vi "AlliGator Phasor Plot Image ROI Storage [SGL] v3.vi"(7 "Current Phasor Plot ROI Color":u32(colorbox), 8 "Error In":errorcluster, 9 "Current ROI Descriptor":T2 {"Contours"."Type" items=["No Selection", "Point", "Line", "Rectangle", "Oval", "Polygon", "Freehand Region", "Annulus", "Unused2", "Unused3", "Broken Line", "Freehand Line", "Rotated Rectangle"]}, 10 "Default Name (\"ROI\")":string="ROI", 11 "Action":T1=enum."Update Current ROI Descriptor") -> (0 "Error Out":errorcluster, 1 "Current ROI Descriptor":T2 {"Contours"."Type" items=["No Selection", "Point", "Line", "Rectangle", "Oval", "Polygon", "Freehand Region", "Annulus", "Unused2", "Unused3", "Broken Line", "Freehand Line", "Rotated Rectangle"]}, 2 "Current ROI Name":string, 3 "Current Phasor Plot Image ROI Index":i32, 4 "Old ROI Name":string, 5 "Current Phasor Plot ROI Color":u32(colorbox))   [LabVIEW 2021, in "AlliGator ROIs.lvlib"]
doc: "Handles single Phasor Plot image ROI storage."
uses:
  AlliGator ROIs.lvlib
  AlliGator ROI Manager Actions.ctl
  Image/Named ROI Description.ctl
  AlliGator Variables List.ctl
  Variant/Variant to Data/Variant to I32.vi
  GUI/GUI.lvlib
  Image/Image.lvlib
  AlliGator Globals, Variables & Constants.lvlib
  Variant/Variant to Data/Variant to Data.lvlib
  Strings/Strings.lvlib
panel:
  # "see the AlliGator License on the block diagram (Ctrl+E or Window:Show Block Diagram)"
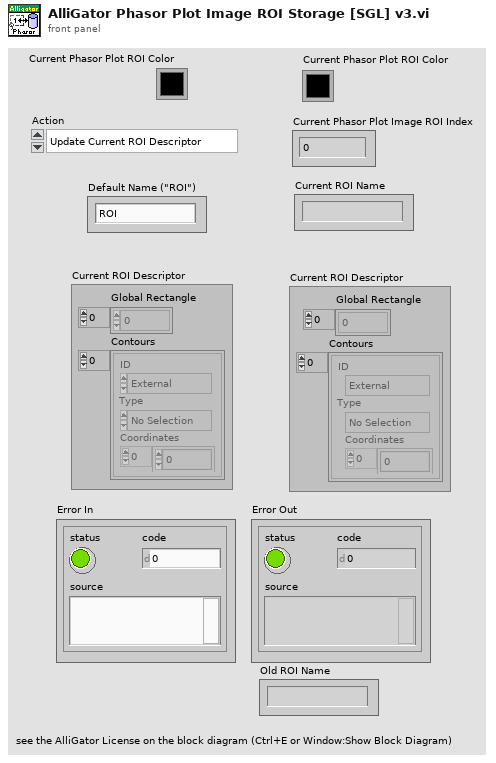
[diagram p1: front panel]
types:
  T1 = typedef "AlliGator ROIs.lvlib/AlliGator ROI Manager Actions.ctl" = enum16{"Undefined", "Delete Current ROI", "Delete All Unselected ROIs", "Delete Multiple ROIs", "Delete All ROIs", "Swap ROIs", "Insert ROI", "Update Current ROI Descriptor", "Rename Current ROI", "Store New ROI", "Store Multiple ROIs", "Select Next ROI", "Select Previous ROI", "Find Selected ROI", "Show All ROIs", "Update ROI Manager Window", "Merge All ROIs", "Unmerge ROI", "Set Selected ROI by ID"}
  T2 = typedef "ROI Descriptor" = cluster{"Global Rectangle":i32[], "Contours":cluster{"ID":enum32{"External", "Internal"}, "Type":u32, "Coordinates":i32[]}[]}
  T3 = typedef "AlliGator Globals, Variables & Constants.lvlib/AlliGator Variables List.ctl" = enum16{"---- GUI ----", "Initialization Status", "State Indicators Refnum", "Original AlliGator Menu Items", "Current Action Loop State", "Script in progress", "Playback", "Loop Playback", "Search ROI Used", "Search ROI", "Decay Graph Max Legend Size", "Intensity Graph Max Legend Size", "Decay Statistics Graph Max Legend Size", "Phasor Graph Max Legend Size", "Phasor Ratio Graph Max Legend Size", "Lifetime Graph Max Legend Size", "---- Files ----", "Export Dataset Frames as Individual Files", "Show Batch Export Help Balloons", "Frames in Dataset", "ptu File Frame Start Indices", "Current Frame in Dataset", "Current Frame Timestamp", "------ Python Plugins ------", "Python Plugins Information", "Python Session", "Valid Python Session?", "---- Source Image ----", "Dataset Loaded", "Dataset Metadata", "Dataset Channel", "Dataset Data Description", "Background Dataset Metadata", "Background Dataset Channel", "Background Dataset Data Description", "Background File Subtraction", "Background File Path", "Background File Pile-up Correction", "Background File Pixel Well Capacity", "Background File Scaling Factor", "Source Image ROIs", "Current Source Image ROI", "Source Image ROI Event Refnum", "X_Source Image Display Range", "X_Source Image Palette Information", "Source Image Palette List", "Source Image Scale", "Current Dataset Load Settings", "Source Image:ROI Overlay Color", "---- Image Profile Window ----", "Image Profile:Overlay ROI in Source Image", "Image Profile Window Event Refnum", "Image Profile:IntensityType", "Image Profile:Intensity Average Type", "Image Profile:Intensity-weighted SDV", "Image Profile:Box Profile Type", "Image Profile Window Open", "Image Profile:Plotted Fit Parameter", "X_Type of Displayed Image", "X_Time Gate Slider", "Dataset Path", "Source Image Overlay to Erase", "Is Displayed Image Accumulated", "White Light Image Modified", "Mask Image Modified", "Macrotime Gate Separation", "------ Phasor Graph -------", "Phasor Graph:Show Line", "---- Phasor Plot ---", "Phasor Plot Parameters Changed", "FLI Dataset Modified since last Phasor Plot Calculation", "Phasor Harmonics Data", "Selected Phasor Harmonics", "Phasor Harmonic Manager Event Refnum", "Phasor Plot ROIs", "Current Phasor Plot ROI", "Phasor Plot ROI Event Refnum", "Phasor Plot Image Reference Points", "Phasor Plot Computed", "Phasor Plot Palette Information", "Phasor Plot Palette List", "Phasor Ratio Palette Information", "Phasor Ratio Palette List", "Phasor Image Scale", "Phasor Plot Image Overlay to Erase", "Phasor Plot Image Elements to Update", "Current Phasor Plot Calculation Parameters", "Current Phasor Calibration Options", "Reset Cumulated Phasor Plot", "Phasor Ratio Reference 1", "Phasor Ratio Lifetime Reference 1", "Phasor Ratio Reference 1 Frequency", "Phasor Ratio Reference 2", "Phasor Ratio Lifetime Reference 2", "Phasor Ratio Reference 2 Frequency", "---- Decay Analysis ----", "Number of Selected Decays to Fit", "LS Fit Results", "LAR Fit Results", "BS Fit Results", "Last Decay Max - Min", "Best Fit Parameters", "Best Fit Parameter Names", "Actual Size X", "Actual Size Y", "Binning X", "Binning Y", "Actual # Gates", "Dataset Number", "Gates to...", "Gates Skipped", "Gates to keep", "Gate Step", "Gate Separation", "Reversed Gates", "Pile-up Correction", "Pixel Well Capacity", "Background Subtracted", "Background Subtraction Method", "Background Definition Range", "Background File (deprecated)", "Number of Dataset Accumulated", "Array of Accumulated Dataset Paths", "Do Averaged Datasets", "Destination File Path", "Process Plot Target", "Use 1/D as Phasor Frequency", "---- Decay Fit Parameter Map -----", "Decay Fit Parameter Map Palette Information", "Decay Fit Parameter Map Palette List", "Local Decay Graph Window Event Refnum", "------- Local Decay Window ---------", "Use normalized IRF for convolution", "----- Miscellaneous ----", "Skippable Dialog Windows Status"}
  T4 = typedef "Image.lvlib/Named ROI Description.ctl" = cluster{"ROI Descriptor":T2, "ROI Name":string, "Overlay Color":u32}
  T5 = typedef "AlliGator ROIs.lvlib/AlliGator Image ROI Event refnum.ctl" = refnum<user-event>
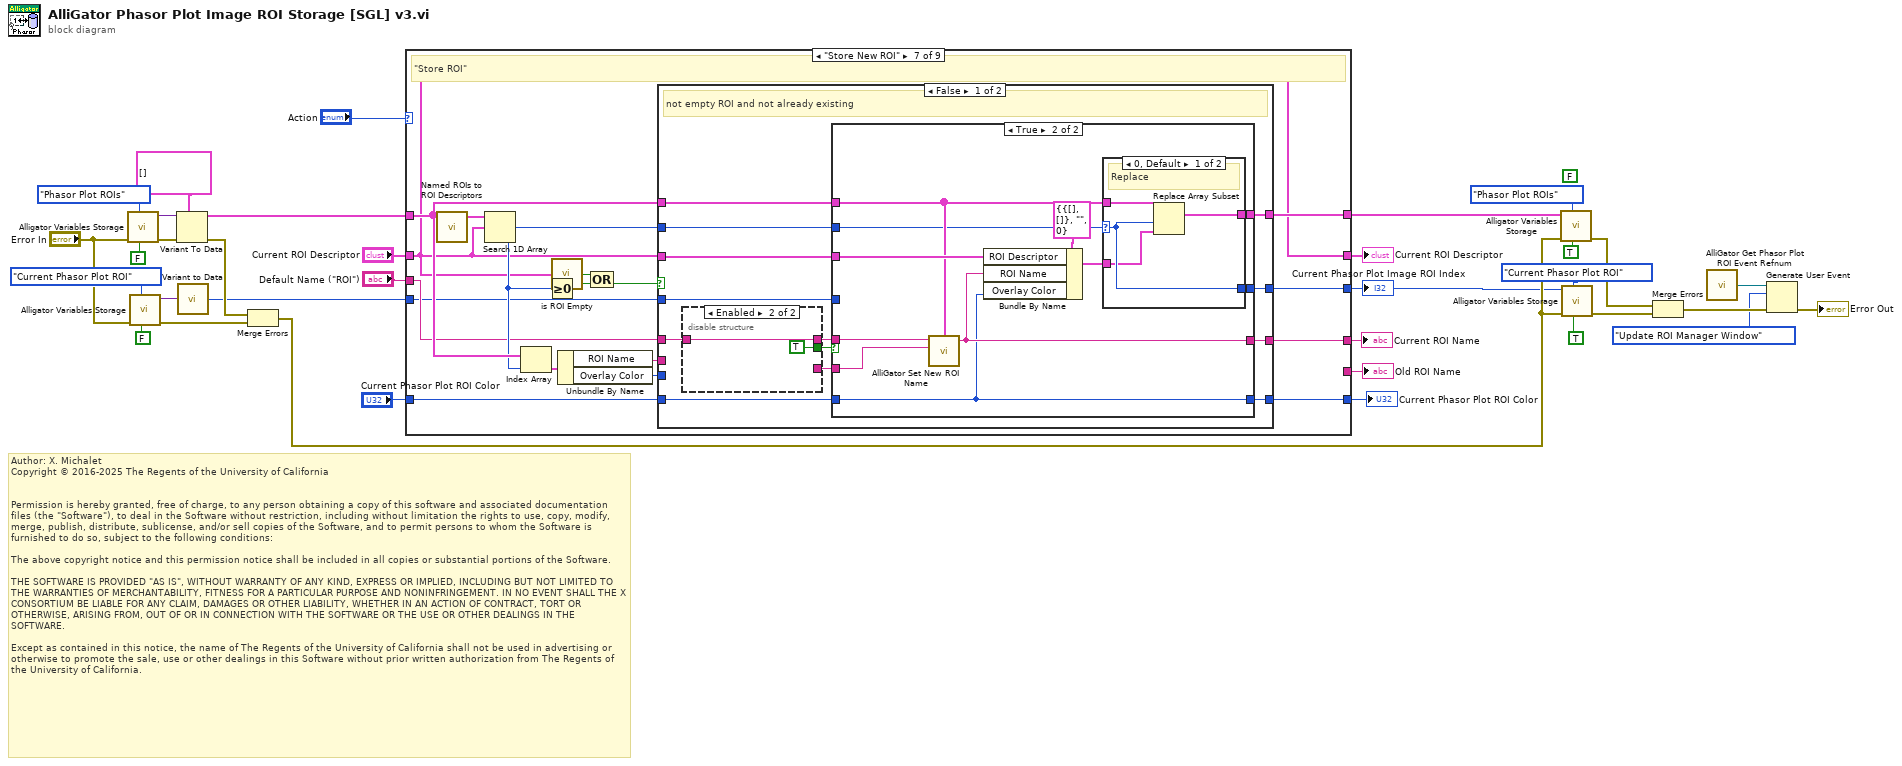
[diagram p0: block diagram]
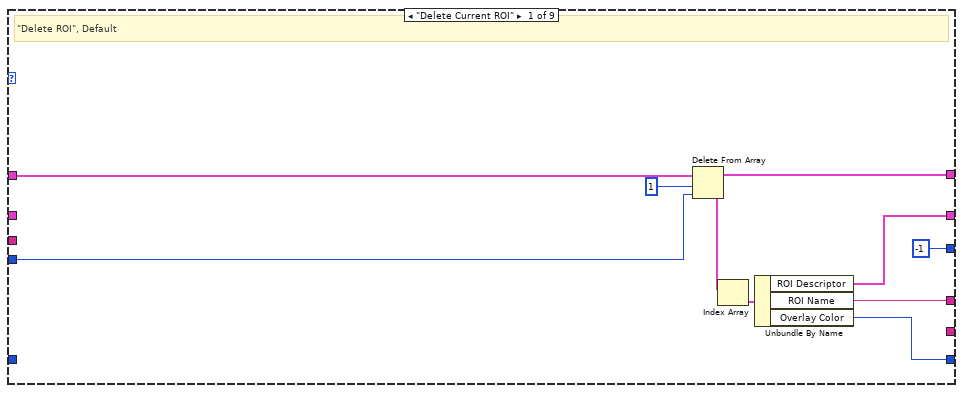
[diagram p2: hidden frame]
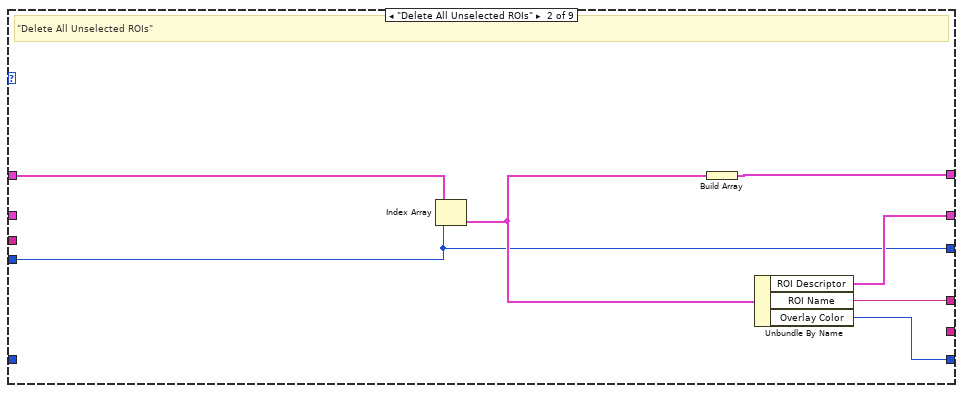
[diagram p3: hidden frame]
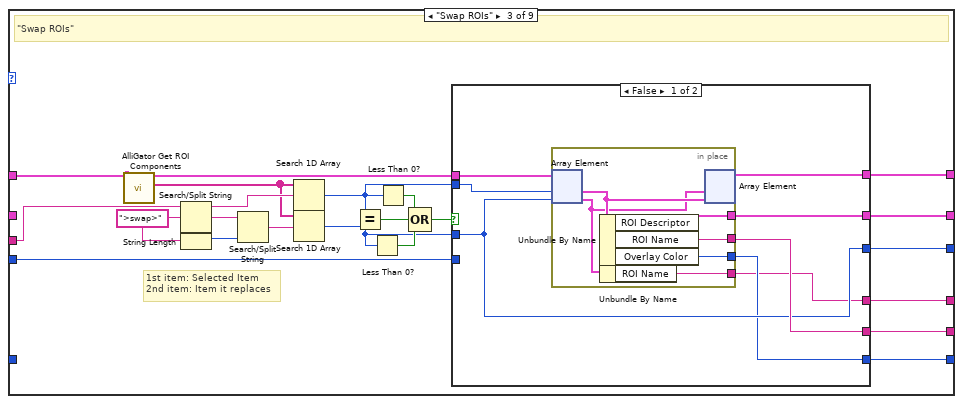
[diagram p4: hidden frame]
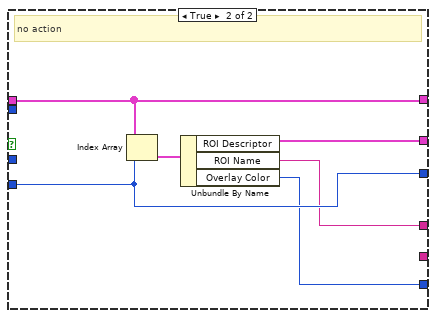
[diagram p5: hidden frame]
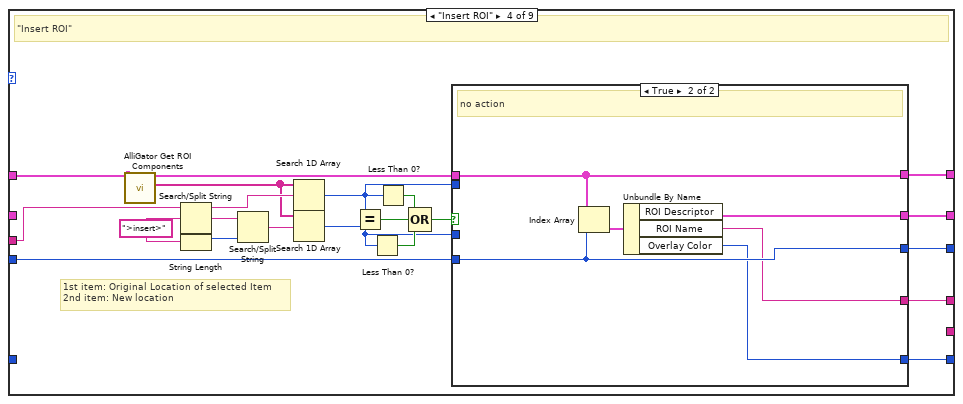
[diagram p6: hidden frame]
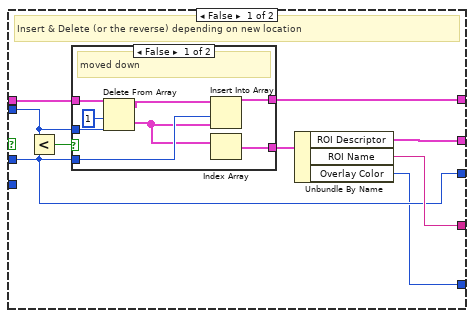
[diagram p7: hidden frame]
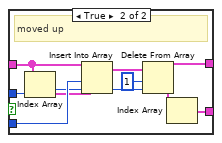
[diagram p8: hidden frame]
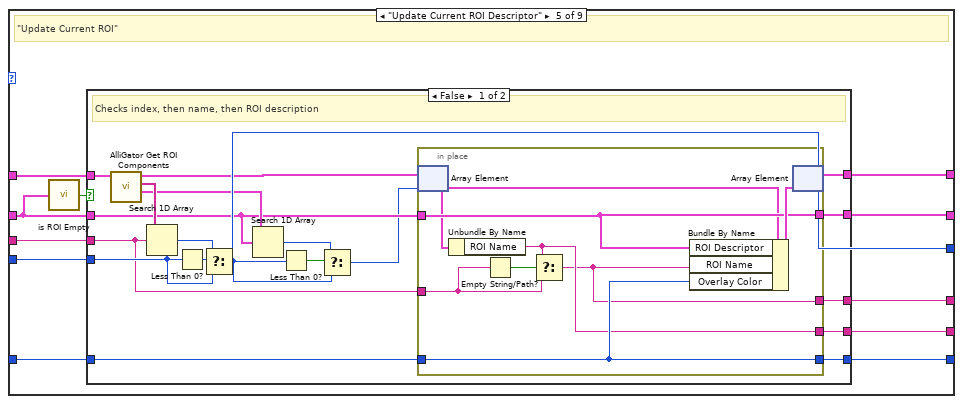
[diagram p9: hidden frame]
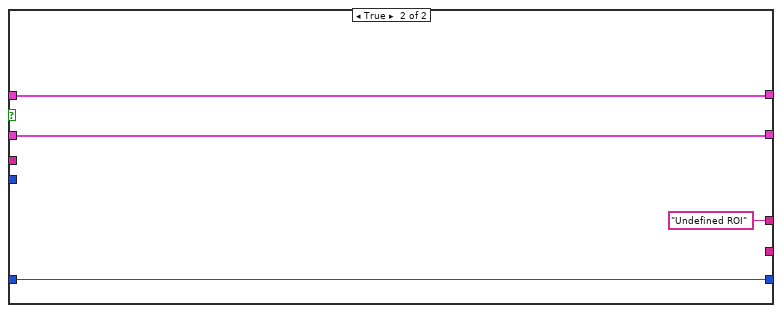
[diagram p10: hidden frame]
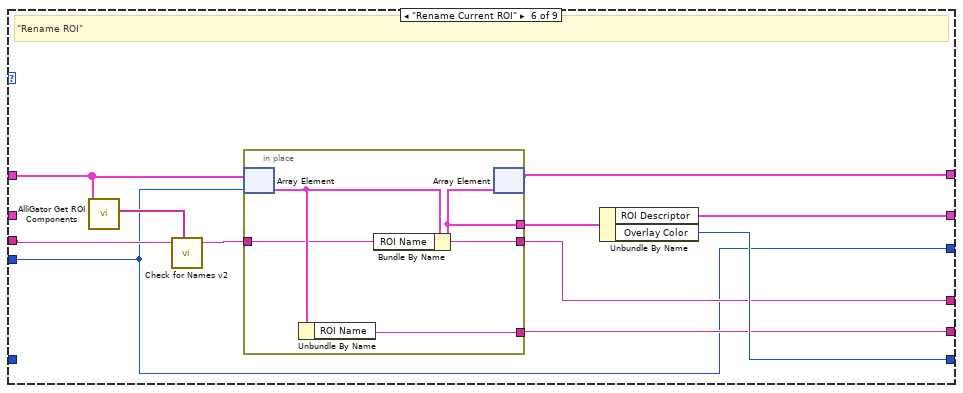
[diagram p11: hidden frame]
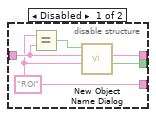
[diagram p12: hidden frame]
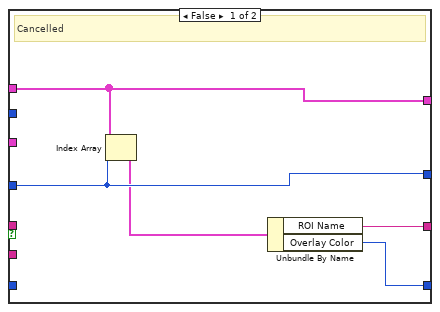
[diagram p13: hidden frame]
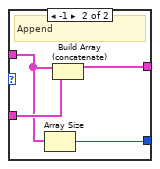
[diagram p14: hidden frame]
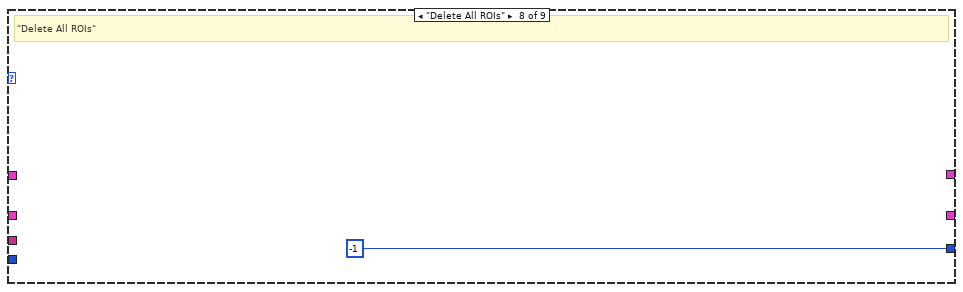
[diagram p16: hidden frame]
diagram:
  (unwired) FALSE ("Get(F)/Set")
  # "Author: X. Michalet\nCopyright © 2016-2025 The Regents of the University of California\n \n\nPermission is hereby granted, free of charge, to any person obtaining a copy of this software and associated documentation files (the \"Software\"), to deal in the Software without restriction, including without limitation the rights to use, copy, modify, merge, publish, distribute, sublicense, and/or sell copies of the Software, and to permit persons to whom the Software is furnished to do so, subject to the following conditions:\n\nThe above copyright notice and this permission notice shall be included in all copies or substantial portions of the Software.\n\nTHE SOFTWARE IS PROVIDED \"AS IS\", WITHOUT WARRANTY OF ANY KIND, EXPRESS OR IMPLIED, INCLUDING BUT NOT LIMITED TO THE WARRANTIES OF MERCHANTABILITY, FITNESS FOR A PARTICULAR PURPOSE AND NONINFRINGEMENT. IN NO EVENT SHALL THE X CONSORTIUM BE LIABLE FOR ANY CLAIM, DAMAGES OR OTHER LIABILITY, WHETHER IN AN ACTION OF CONTRACT, TORT OR OTHERWISE, ARISING FROM, OUT OF OR IN CONNECTION WITH THE SOFTWARE OR THE USE OR OTHER DEALINGS IN THE SOFTWARE.\n\nExcept as contained in this notice, the name of The Regents of the University of California shall not be used in advertising or otherwise to promote the sale, use or other dealings in this Software without prior written authorization from The Regents of the University of California."
  n1 = call "Alligator Variables Storage.vi"("Get(F)/Set"=FALSE, "AlliGator Variable"=AlliGator_Variables_List."Phasor Plot ROIs" ("Alligator Variable"), "Error In"="Error In") -> ("Error Out"=w32:errorcluster, "Data out"=w33:variant)  [unwired: 6 in, 1 out]
  n2 = call "Alligator Variables Storage.vi"("Get(F)/Set"=FALSE, "AlliGator Variable"=AlliGator_Variables_List."Current Phasor Plot ROI" ("Alligator Variable"), "Error In"="Error In") -> ("Error Out"=w22:errorcluster, "Data out"=w27:variant)  [unwired: 6 in, 1 out]
  n3 = Variant To Data(error in=w32, type=T4[] [] ("Stored ROIs in"), Variant=w33) -> (data=w14:T4[], error out=w21:errorcluster)
  n4 = call-poly "Variant to Data.vi"("Variant"=w27) -> ("Value"=w13:i32)  [unwired: 8 in]
  n5 = Merge Errors(w21, w22) -> (w15:errorcluster)
  n6 = case shown="\"Store New ROI\"" "Action" {
    tunnel: w14 -> [w44 w48 w52 w93 w155 w191 w214 _ w268]
    tunnel: w13 -> [w43 w45 w72 w112 w152 w186 w201 _ w267]
    tunnel: [w41 w47 w71 w111 w154 w190 w217 _ w268] -> w10
    tunnel: [-1 ("Current ROI out") w45 w70 w110 w152 w186 w216 -1 ("index of element") w267] -> w9
    tunnel: "Current ROI Descriptor" -> [_ _ _ _ w151 _ w208 _ w270]
    tunnel: [w36 w50 w57 w98 w153 w196 w208 _ w270] -> w8
    tunnel: "Default Name (\"ROI\")" -> [_ _ w68 w109 w145 w192 w209 _ _]
    tunnel: [w35 w49 w56 w97 w149 w188 w205 _ _] -> w7
    tunnel: [_ _ w69 _ w146 w187 _ _ _] -> w6
    tunnel: [w37 w51 w53 w94 w148 w195 w202 _ w269] -> w5
    tunnel: "Current Phasor Plot ROI Color" -> [_ _ _ _ w147 _ w203 _ w269]
    frame "Delete Current ROI" {
      # "\"Delete ROI\", Default"
      n7 = Delete From Array(array=w44, length=1, index=w43) -> (deleted portion=w39:T4[], array with subset deleted=w41:T4[])
      n8 = Index Array(array=w39) -> (element=w38:T4)  [unwired: 1 in]
      n9 = Unbundle By Name(w38) -> ("ROI Descriptor"=w36:T2, "ROI Name"=w35:string, "Overlay Color"=w37:u32)
    }
    frame "Delete All Unselected ROIs" {
      # "\"Delete All Unselected ROIs\""
      n10 = Index Array(array=w48, index=w45) -> (element=w46:T4)
      n11 = Build Array(w46) -> (w47:T4[])
      n12 = Unbundle By Name(w46) -> ("ROI Descriptor"=w50:T2, "ROI Name"=w49:string, "Overlay Color"=w51:u32)
    }
    frame "Swap ROIs" {
      w66 = ">swap>" ("search string/char (-)")
      # "1st item: Selected Item\n2nd item: Item it replaces"
      # "\"Swap ROIs\""
      n13 = call "AlliGator Get ROI Components.vi"("Stored ROIs"=w52) -> ("ROI Names"=w63:string[])  [unwired: 8 in, 2 out]
      n14 = Search/Split String(string=w68, search string/char (-)=w66) -> (substring before match=w64:string, match + rest of string=w67:string)  [unwired: 1 in, 1 out]
      n15 = String Length(string=w66) -> (length=w65:i32)
      n16 = Search/Split String(string=w67, offset (0)=w65) -> (match + rest of string=w62:string)  [unwired: 1 in, 2 out]
      n17 = Search 1D Array(1D array=w63, element=w64) -> (index of element=w55:i32)  [unwired: 1 in]
      n18 = Search 1D Array(1D array=w63, element=w62) -> (index of element=w54:i32)  [unwired: 1 in]
      n19 = Equal?(x=w55, y=w54) -> (x = y?=w59:bool)
      n20 = Less Than 0?(x=w54) -> (x < 0?=w60:bool)
      n21 = Less Than 0?(x=w55) -> (x < 0?=w61:bool)
      n22 = Compound Arithmetic op=OR(w61, w59, w60) -> (w58:bool)
      n23 = case shown="False" w58 {
        tunnel: w72 -> [_ w91]
        tunnel: [w79 w92] -> w71
        tunnel: [w75 w91] -> w70
        tunnel: [w76 _] -> w69
        tunnel: w52 -> [w80 w92]
        tunnel: [w77 w89] -> w57
        tunnel: [w73 w88] -> w56
        tunnel: w55 -> [w78 _]
        tunnel: w54 -> [w75 _]
        tunnel: [w74 w87] -> w53
        frame False {
          n24 = in-place {
            in-place-border: [w85] -> w77
            in-place-border: [w84] -> w76
            in-place-border: [w83] -> w74
            in-place-border: [w81] -> w73
            n25 = in-place-array #1(w80, w78, w75) -> (w86:T4, w82:T4)
            n26 = Unbundle By Name(w86) -> ("ROI Descriptor"=w85:T2, "ROI Name"=w84:string, "Overlay Color"=w83:u32)
            n27 = Unbundle By Name(w82) -> ("ROI Name"=w81:string)
            n28 = in-place-array #1(w82, w86) -> (w79:T4[])  [unwired: 2 out]
          }
        }
        frame True {
          # "no action"
          n29 = Index Array(array=w92, index=w91) -> (element=w90:T4)
          n30 = Unbundle By Name(w90) -> ("ROI Descriptor"=w89:T2, "ROI Name"=w88:string, "Overlay Color"=w87:u32)
        }
      }
    }
    frame "Insert ROI" {
      w107 = ">insert>" ("search string/char (-)")
      # "1st item: Original Location of selected Item\n2nd item: New location"
      # "\"Insert ROI\""
      n31 = call "AlliGator Get ROI Components.vi"("Stored ROIs"=w93) -> ("ROI Names"=w104:string[])  [unwired: 8 in, 2 out]
      n32 = Search/Split String(string=w109, search string/char (-)=w107) -> (substring before match=w105:string, match + rest of string=w108:string)  [unwired: 1 in, 1 out]
      n33 = String Length(string=w107) -> (length=w106:i32)
      n34 = Search/Split String(string=w108, offset (0)=w106) -> (match + rest of string=w103:string)  [unwired: 1 in, 2 out]
      n35 = Search 1D Array(1D array=w104, element=w105) -> (index of element=w96:i32)  [unwired: 1 in]
      n36 = Search 1D Array(1D array=w104, element=w103) -> (index of element=w95:i32)  [unwired: 1 in]
      n37 = Equal?(x=w96, y=w95) -> (x = y?=w100:bool)
      n38 = Less Than 0?(x=w95) -> (x < 0?=w101:bool)
      n39 = Less Than 0?(x=w96) -> (x < 0?=w102:bool)
      n40 = Compound Arithmetic op=OR(w102, w100, w101) -> (w99:bool)
      n41 = case shown="True" w99 {
        tunnel: w112 -> [_ w143]
        tunnel: [w118 w144] -> w111
        tunnel: [w114 w143] -> w110
        tunnel: w93 -> [w120 w144]
        tunnel: [w116 w141] -> w98
        tunnel: [w115 w140] -> w97
        tunnel: w96 -> [w119 _]
        tunnel: w95 -> [w114 _]
        tunnel: [w113 w139] -> w94
        frame False {
          # "Insert & Delete (or the reverse) depending on new location"
          n42 = Less?(x=w119, y=w114) -> (x < y?=w121:bool)
          n43 = case shown="False" w121 {
            tunnel: w120 -> [w129 w138]
            tunnel: w119 -> [w128 w134]
            tunnel: w114 -> [w124 w137]
            tunnel: [w125 w132] -> w118
            tunnel: [w122 w130] -> w117
            frame False {
              # "moved down"
              n44 = Delete From Array(array=w129, length=1, index=w128) -> (deleted portion=w123:T4[], array with subset deleted=w126:T4[])
              n45 = Insert Into Array(array=w126, index=w124, new element=w123) -> (w125:T4[])
              n46 = Index Array(array=w123) -> (element=w122:T4)  [unwired: 1 in]
            }
            frame True {
              # "moved up"
              n47 = Index Array(array=w138, index=w134) -> (element=w136:T4)
              n48 = Insert Into Array(array=w138, index=w137, new element=w136) -> (w135:T4[])
              n49 = Delete From Array(array=w135, length=1, index=w134) -> (deleted portion=w131:T4[], array with subset deleted=w132:T4[])
              n50 = Index Array(array=w131) -> (element=w130:T4)  [unwired: 1 in]
            }
          }
          n51 = Unbundle By Name(w117) -> ("ROI Descriptor"=w116:T2, "ROI Name"=w115:string, "Overlay Color"=w113:u32)
        }
        frame True {
          # "no action"
          n52 = Index Array(array=w144, index=w143) -> (element=w142:T4)
          n53 = Unbundle By Name(w142) -> ("ROI Descriptor"=w141:T2, "ROI Name"=w140:string, "Overlay Color"=w139:u32)
        }
      }
    }
    frame "Update Current ROI Descriptor" {
      # "\"Update Current ROI\""
      n54 = call "is ROI Empty.vi"("Current ROI Descriptor"=w151) -> ("Empty ROI?"=w150:bool)  [unwired: 8 in]
      n55 = case shown="False" w150 {
        tunnel: w155 -> [w166 w185]
        tunnel: [w173 w185] -> w154
        tunnel: [w172 w184] -> w153
        tunnel: [w156 "Undefined ROI" ("ROI Name")] -> w149
        tunnel: w152 -> [w167 _]
        tunnel: w151 -> [w162 w184]
        tunnel: [w169 w182] -> w148
        tunnel: w147 -> [w170 w182]
        tunnel: [w171 _] -> w146
        tunnel: w145 -> [w157 _]
        frame False {
          # "Checks index, then name, then ROI description"
          n56 = call "AlliGator Get ROI Components.vi"("Stored ROIs"=w166) -> ("ROI Descriptors"=w163:T2[], "ROI Names"=w165:string[])  [unwired: 8 in, 1 out]
          n57 = Search 1D Array(1D array=w165, element=w157) -> (index of element=w164:i32)  [unwired: 1 in]
          n58 = Less Than 0?(x=w167) -> (x < 0?=w168:bool)
          n59 = Select(t=w164, s=w168, f=w167) -> (s? t:f=w159:i32)
          n60 = Search 1D Array(1D array=w163, element=w162) -> (index of element=w160:i32)  [unwired: 1 in]
          n61 = Less Than 0?(x=w159) -> (x < 0?=w161:bool)
          n62 = Select(t=w160, s=w161, f=w159) -> (s? t:f=w158:i32)
          n63 = in-place {
            in-place-border: w162 -> [w180]
            in-place-border: [w180] -> w172
            in-place-border: [w176] -> w171
            in-place-border: w170 -> [w179]
            in-place-border: [w179] -> w169
            in-place-border: w157 -> [w175]
            in-place-border: [w174] -> w156
            n64 = in-place-array #2(w166, w158) -> (w177:T4)
            n65 = Unbundle By Name(w177) -> ("ROI Name"=w176:string)
            n66 = Empty String/Path?(string/path=w175) -> (empty?=w178:bool)
            n67 = Select(t=w176, s=w178, f=w175) -> (s? t:f=w174:string)
            n68 = Bundle By Name(cluster=w177, "ROI Descriptor"=w180, "ROI Name"=w174, "Overlay Color"=w179) -> (w181:T4)
            n69 = in-place-array #2(w181) -> (w173:T4[])  [unwired: 1 out]
          }
        }
        frame True {
        }
      }
    }
    frame "Rename Current ROI" {
      # "\"Rename ROI\""
      n70 = call "AlliGator Get ROI Components.vi"("Stored ROIs"=w191) -> ("ROI Names"=w194:string[])  [unwired: 8 in, 2 out]
      n71 = call "Check for Names v2.vi"("New Name"=w192, "Name List"=w194) -> ("New Name"=w193:string)  [unwired: 4 in, 3 out]
      n72 = in-place {
        in-place-border: w193 -> [w197]
        in-place-border: [w200] -> w189
        in-place-border: [w198] -> w187
        in-place-border: [w197] -> w188
        n73 = in-place-array #3(w191, w186) -> (w199:T4)
        n74 = Unbundle By Name(w199) -> ("ROI Name"=w198:string)
        n75 = Bundle By Name(cluster=w199, "ROI Name"=w197) -> (w200:T4)
        n76 = in-place-array #3(w200) -> (w190:T4[])  [unwired: 1 out]
      }
      n77 = Unbundle By Name(w189) -> ("ROI Descriptor"=w196:T2, "Overlay Color"=w195:u32)
    }
    frame "Store New ROI" {
      # "\"Store ROI\""
      n78 = call "Named ROIs to ROI Descriptors.vi"("Named ROIs"=w214) -> ("ROI Descriptors"=w215:T2[])  [unwired: 10 in]
      n79 = Search 1D Array(1D array=w215, element=w208) -> (index of element=w211:i32)  [unwired: 1 in]
      n80 = Index Array(array=w214, index=w211) -> (element=w213:T4)
      n81 = Greater Or Equal To 0?(x=w211) -> (x >= 0?=w210:bool)
      n82 = call "is ROI Empty.vi"("Current ROI Descriptor"=w208) -> ("Empty ROI?"=w206:bool)  [unwired: 8 in]
      n83 = Unbundle By Name(w213) -> ("ROI Name"=w212:string, "Overlay Color"=w204:u32)
      n84 = Compound Arithmetic op=OR(w206, w210) -> (w207:bool)
      n85 = case shown="False" w207 {
        tunnel: [w230 w265] -> w217
        tunnel: [w229 w263] -> w216
        tunnel: w208 -> [w228 _]
        tunnel: w214 -> [w227 w265]
        tunnel: w212 -> [_ w264]
        tunnel: w211 -> [w226 w263]
        tunnel: w209 -> [w223 _]
        tunnel: [w224 w264] -> w205
        tunnel: w204 -> [_ w262]
        tunnel: w203 -> [w218 _]
        tunnel: [w219 w262] -> w202
        tunnel: w201 -> [w220 _]
        frame False {
          # "not empty ROI and not already existing"
          n86 = disable-structure shown="Enabled" {
            disable-tunnel: [w235 w237] -> w225
            disable-tunnel: w223 -> [w233 w237]
            disable-tunnel: [w232 _] -> w222
            disable-tunnel: [w231 TRUE ("OK")] -> w221
            frame Disabled {
              w232 = "ROI" ("x")
              n87 = Equal?(x=w232, y=w233) -> (x = y?=w234:bool)
              n88 = call "New Object Name Dialog.vi"("String Name (\"object\")"=w232, "Object Name in"=w233, "Enable"=w234) -> ("OK"=w231:bool, "Object Name out"=w235:string)  [unwired: 6 in, 1 out]
            }
            frame Enabled {
            }
          }
          n89 = case shown="True" w221 {
            tunnel: [w242 w253] -> w230
            tunnel: [w241 w252] -> w229
            tunnel: w228 -> [_ w249]
            tunnel: w227 -> [w242 w248]
            tunnel: w226 -> [_ w247]
            tunnel: w225 -> [_ w246]
            tunnel: [w239 w245] -> w224
            tunnel: w222 -> [_ w244]
            tunnel: w220 -> [w241 _]
            tunnel: [w238 w243] -> w219
            tunnel: w218 -> [_ w243]
            frame False {
              # "Cancelled"
              n90 = Index Array(array=w242, index=w241) -> (element=w240:T4)
              n91 = Unbundle By Name(w240) -> ("ROI Name"=w239:string, "Overlay Color"=w238:u32)
            }
            frame True {
              n92 = call "AlliGator Set New ROI Name.vi"("Stored ROIs in"=w248, "ROI Name in"=w246, "Default Name (\"\")"=w244) -> ("ROI Name out"=w245:string)  [unwired: 6 in]
              n93 = Bundle By Name(cluster=T4 {"ROI Descriptor"={"Global Rectangle"=[], "Contours"=[]}, "ROI Name"="", "Overlay Color"=0} ("Named ROI Description"), "ROI Descriptor"=w249, "ROI Name"=w245, "Overlay Color"=w243) -> (w250:T4)
              n94 = case shown="0, Default" w247 {
                selector: w247 -> [w256 _]
                tunnel: [w255 w261] -> w253
                tunnel: [w256 w260] -> w252
                tunnel: w250 -> [w254 w259]
                tunnel: w248 -> [w257 w258]
                frame 0, Default {
                  # "Replace"
                  n95 = Replace Array Subset(array=w257, new element=w254, index=w256) -> (w255:T4[])
                }
                frame -1 {
                  # "Append"
                  n96 = Array Size(array=w258) -> (size(s)=w260:i32)
                  n97 = Build Array (concatenate)(w258, w259) -> (w261:T4[])
                }
              }
            }
          }
        }
        frame True {
          # "no need to change or empty ROI"
        }
      }
    }
    frame "Delete All ROIs" {
      # "\"Delete All ROIs\""
    }
    frame Default {
    }
  }
  "Current ROI Descriptor" <- w8
  "Current Phasor Plot Image ROI Index" <- w9
  "Current ROI Name" <- w7
  "Old ROI Name" <- w6
  "Current Phasor Plot ROI Color" <- w5
  n98 = call "Alligator Variables Storage.vi"("Get(F)/Set"=TRUE, "AlliGator Variable"=AlliGator_Variables_List."Phasor Plot ROIs" ("Alligator Variable"), "Error In"=w15, "Data in"=w10) -> ("Error Out"=w19:errorcluster)  [unwired: 5 in, 2 out]
  n99 = call "Alligator Variables Storage.vi"("Get(F)/Set"=TRUE, "AlliGator Variable"=AlliGator_Variables_List."Current Phasor Plot ROI" ("Alligator Variable"), "Error In"=w15, "Data in"=w9) -> ("Error Out"=w20:errorcluster)  [unwired: 5 in, 2 out]
  n100 = Merge Errors(w19, w20) -> (w17:errorcluster)
  n101 = call "AlliGator Get Phasor Plot ROI Event Refnum.vi"() -> ("Phasor Plot ROI Event Refnum"=w2:T5)
  n102 = Generate User Event(user event=w2, event data cluster=AlliGator_ROI_Manager_Actions."Update ROI Manager Window" ("event data"), error in=w17) -> (error out=→"Error Out":errorcluster)  [unwired: 1 in, 1 out]
